vi "CRYStatistics.vi"(0 "Setup in":T1={"No.VI"=0, "Category"="", "StepName"="", "Seq setup flattened"="", "Comment"="", "Steps config."=[], "Jump config"=[], "Start"=0.0, "Increment"=0.0, "Name"="Pa", "Unit"="Pa", "Y data"=1, "Y prefix"="", "Y dB ref"=1.0, "Y unit"="", "Repeat State Array"=[]} {"Repeat State Array"."Start" format="%#_5g"; "Y dB ref" format="%.1f"; "Y data" items=["dB", "Lin"]; "Start" format="%#_5g"}, 5 "Data in":T6 {"Z data" items=["dB", "Lin"]; "X data" items=["dB", "Lin"]; "Y data" items=["dB", "Lin"]; "Z dB ref" format="%.1f"; "Z axis" items=["Log", "Lin"]; "X dB ref" format="%.1f"; "X axis" items=["Log", "Lin"]; "Y axis" items=["Log", "Lin"]; "Y dB ref" format="%.1f"; "Curve"."z" format="%.2f"; "Curve"."y" format="%.2f"; "Curve"."x" format="%.2f"}, 7 "Results in":T2 {"Margin" format="%.2f"}, 9 "Seq Setup in":string, 11 "Step name":string, 12 "Hardware in":string, 13 "Calibration in":string) -> (3 "Types Out":string[](array[string]), 4 "Inserted Names Out":string[](array[string]), 6 "Data out":T6 {"Z data" items=["dB", "Lin"]; "X data" items=["dB", "Lin"]; "Y data" items=["dB", "Lin"]; "Z dB ref" format="%.1f"; "Z axis" items=["Log", "Lin"]; "X dB ref" format="%.1f"; "X axis" items=["Log", "Lin"]; "Y axis" items=["Log", "Lin"]; "Y dB ref" format="%.1f"; "Curve"."z" format="%.2f"; "Curve"."y" format="%.2f"; "Curve"."x" format="%.2f"}, 8 "Results out":T2 {"Margin" format="%.2f"}, 10 "Wave out":T4 {"Y dB ref" format="%.1f"; "Y axis" items=["Log", "Lin"]; "Y data" items=["dB", "Lin"]; "X data" items=["dB", "Lin"]})   [LabVIEW 2013]
uses:
  Typedef Control/CRYData Cluster Array.ctl
  Typedef Control/CRYData Cluster.ctl
  Typedef Control/CRYResult Cluster Array.ctl
  Typedef Control/CRYResult Cluster.ctl
  Typedef Control/CRYWaveform Cluster Array.ctl
  Typedef Control/CRYWaveform Cluster.ctl
  Typedef Control/CRYStep.ctl
  Task Sequence/CRYProject Run Control Global.vi
panel:
  in  "Display Step":bool=TRUE
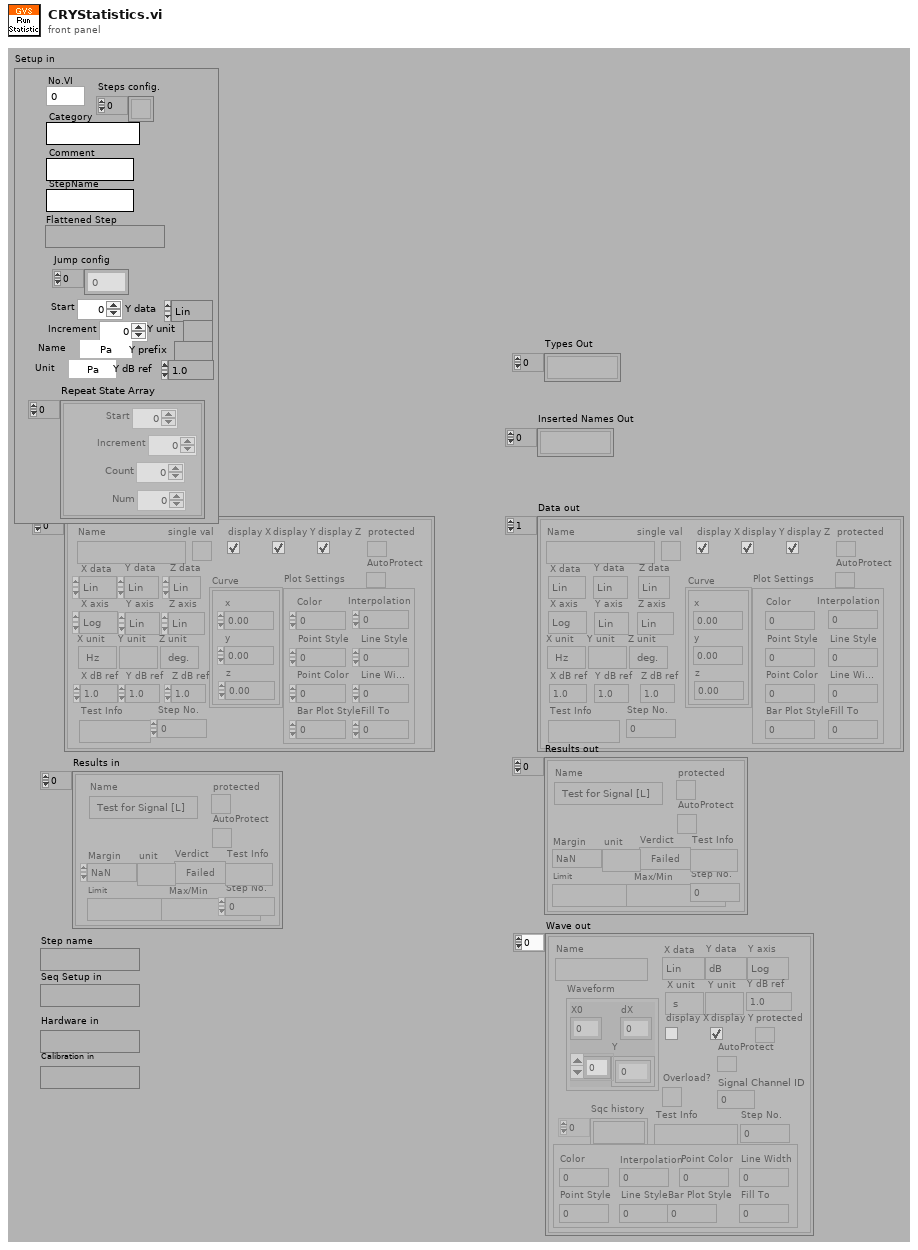
[diagram p1: front panel]
types:
  T1 = typedef "CRYStep.ctl" = cluster{"No.VI":i32, "Category":string, "StepName":string, "Seq setup flattened":string, "Comment":string, "Steps config.":bool[], "Jump config":i32[], "Start":dbl, "Increment":dbl, "Name":string, "Unit":string, "Y data":u16, "Y prefix":string, "Y dB ref":dbl, "Y unit":string, "Repeat State Array":cluster{"Start":dbl, "Increment":dbl, "Count":i32, "Num":i32}[]}
  T2 = typedef "CRYResult Cluster Array.ctl" = T3[]
  T3 = typedef "CRYResult Cluster.ctl" = cluster{"Name":string, "Margin":dbl, "unit":string, "Verdict":bool, "Limit":string, "Max/Min":string, "protected":bool, "Step No.":i32, "Test Info":string, "AutoProtect":bool}
  T4 = typedef "CRYWaveform Cluster Array.ctl" = T5[]
  T5 = typedef "CRYWaveform Cluster.ctl" = cluster{"Waveform":cluster{"X0":dbl, "dX":dbl, "Y":sgl[]}, "X data":u16, "Y data":u16, "Y axis":u16, "X unit":string, "Y unit":string, "Y dB ref":dbl, "display Y":bool, "display X":bool, "Overload?":bool, "Test Info":string, "Step No.":i32, "Name":string, "protected":bool, "Sqc history":string[], "Signal Channel ID":i32, "Plot Settings":cluster{"Color":u32, "Interpolation":u8, "Point Style":u8, "Line Style":u8, "Point Color":u32, "Line Width":u8, "Bar Plot Style":u8, "Fill To":i16}, "AutoProtect":bool}
  T6 = typedef "CRYData Cluster Array.ctl" = T7[]
  T7 = typedef "CRYData Cluster.ctl" = cluster{"Name":string, "Curve":cluster{"x":dbl, "y":dbl, "z":dbl}[], "X data":u16, "Y data":u16, "Z data":u16, "X axis":u16, "Y axis":u16, "Z axis":u16, "X unit":string, "Y unit":string, "Z unit":string, "X dB ref":dbl, "Y dB ref":dbl, "Z dB ref":dbl, "single val":bool, "protected":bool, "display X":bool, "display Y":bool, "display Z":bool, "Test Info":string, "Step No.":i32, "Plot Settings":cluster{"Color":u32, "Interpolation":u8, "Point Style":u8, "Line Style":u8, "Point Color":u32, "Line Width":u8, "Bar Plot Style":u8, "Fill To":i16}, "AutoProtect":bool}
  T8 = cluster{"Start":dbl, "Increment":dbl, "Count":i32, "Num":i32}[]
  T9 = typedef "CRYStatistic cluster.ctl" = cluster{"Mode":u16, "No.Ranked(BF)":i32, "No.Ranked(WF)":i32, "Absolute Margin Standard Deviation":bool, "+/- sigma Res":i32, "Margin Standard Deviation":bool, "Margin Mean":bool, "Overall Yield":bool, "Individual Limits Yield":bool, "LSL Unit":string, "USL Unit\n":string, "LSL":dbl, "USL":dbl, "Worst Fit to Average":bool, "Best Fit to Average":bool, "Ppk":bool, "Pp":bool, "Absolute Standard Deviation":bool, "+/- sigma Dat":i32, "Standard Deviation ":bool, "Mean":bool, "Min ":bool, "Max ":bool, "No.of Curves Selected":i32, "Curves":string[], " Results":string[], "Name":string, "Help":string, "Tab Value":enum32{"Setting", "Help"}, "Work in":u16, "Mode xyz":u16}
  T10 = cluster{"Max ":bool, "Min ":bool, "Mean":bool, "Absolute Standard Deviation":bool, "Standard Deviation ":bool, "Pp":bool, "Ppk":bool, "Best Fit to Average":bool, "Worst Fit to Average":bool}
  T11 = cluster{"Individual Limits Yield":bool, "Overall Yield":bool, "Margin Mean":bool, "Absolute Margin Standard Deviation":bool, "Margin Standard Deviation":bool}
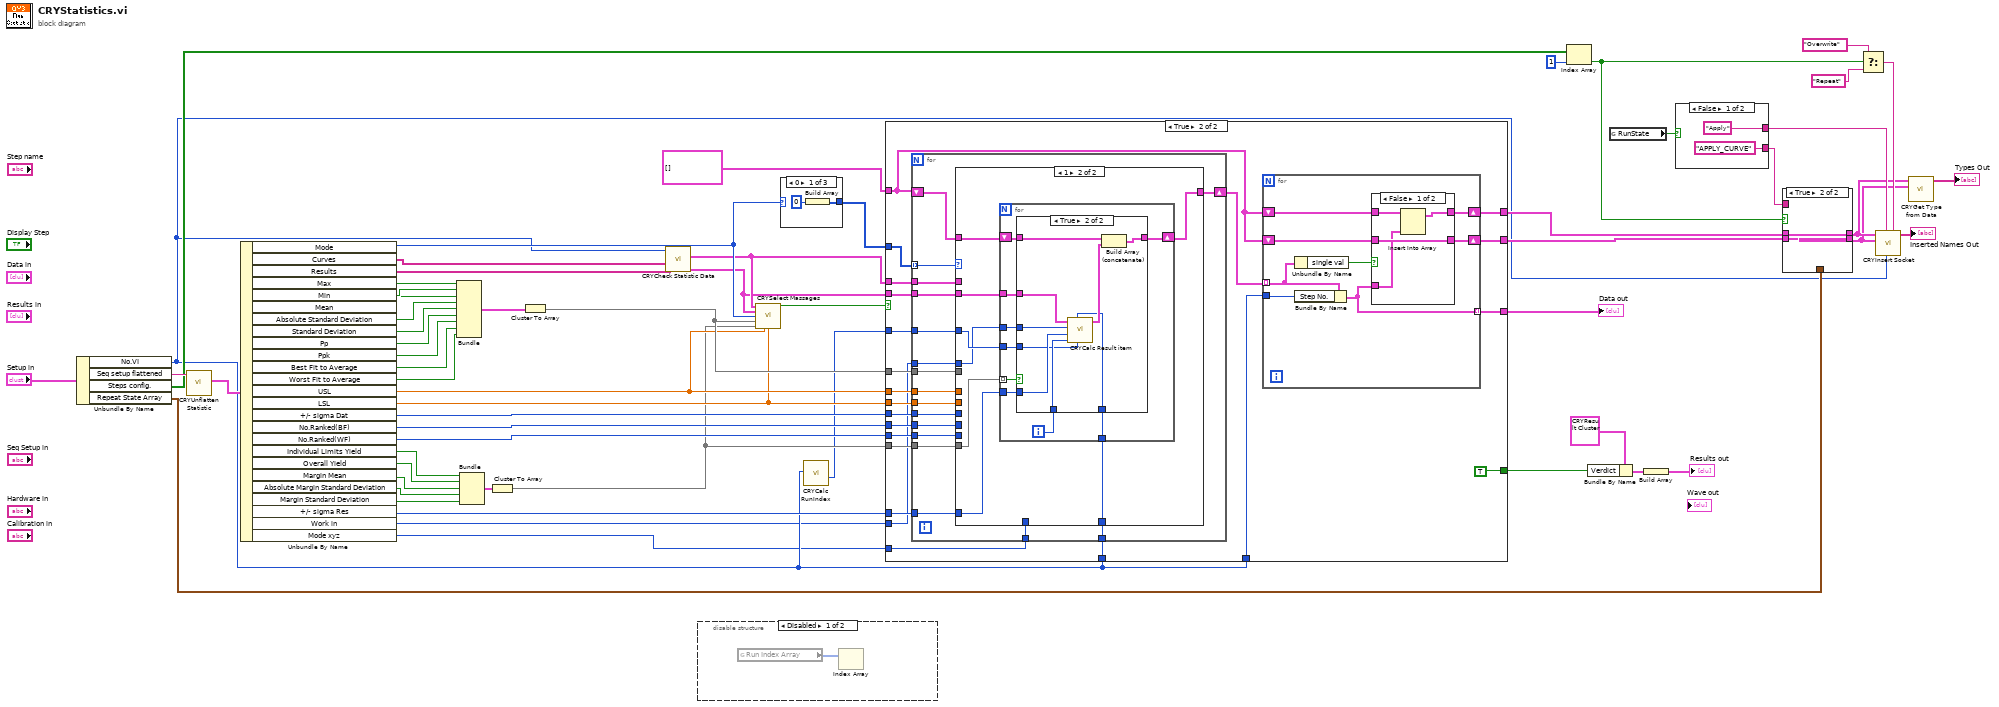
[diagram p0: block diagram]
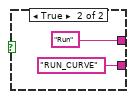
[diagram p3: hidden frame]
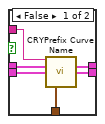
[diagram p4: hidden frame]
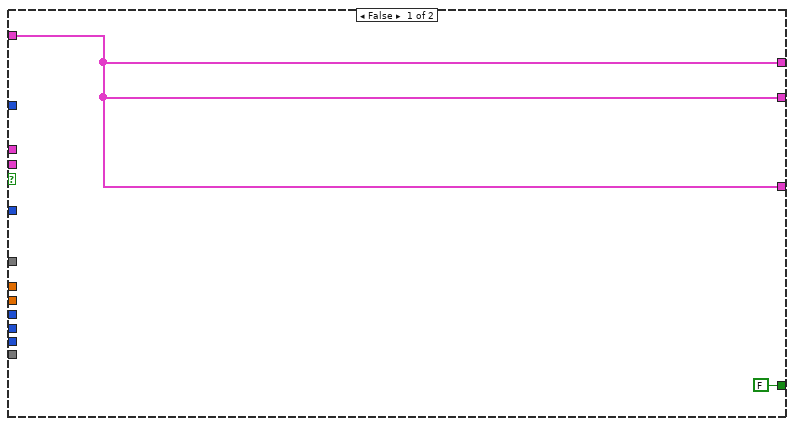
[diagram p5: hidden frame]
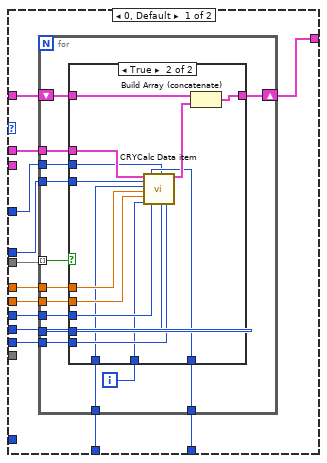
[diagram p6: hidden frame]
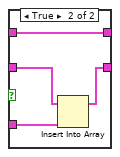
[diagram p9: hidden frame]
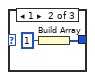
[diagram p10: hidden frame]
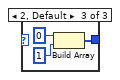
[diagram p11: hidden frame]
diagram:
  n1 = Unbundle By Name("Setup in") -> ("No.VI"=w3:i32, "Seq setup flattened"=w27:string, "Steps config."=w22:bool[], "Repeat State Array"=w17:T8)
  n2 = call "CRYUnflatten Statistic.vi"("Flatten Statistics"=w27) -> ("Statistics"=w29:T9)  [unwired: 10 out]
  n3 = Unbundle By Name(w29) -> ("Mode"=w52:u16, "Curves"=w7:string[], "Results"=w6:string[], "Max"=w44:bool, "Min"=w43:bool, "Mean"=w42:bool, "Absolute Standard Deviation"=w41:bool, "Standard Deviation"=w40:bool, "Pp"=w39:bool, "Ppk"=w38:bool, "Best Fit to Average"=w37:bool, "Worst Fit to Average"=w36:bool, "USL"=w55:dbl, "LSL"=w54:dbl, "+/- sigma Dat"=w60:i32, "No.Ranked(BF)"=w59:i32, "No.Ranked(WF)"=w58:i32, "Individual Limits Yield"=w34:bool, "Overall Yield"=w33:bool, "Margin Mean"=w32:bool, "Absolute Margin Standard Deviation"=w31:bool, "Margin Standard Deviation"=w30:bool, "+/- sigma Res"=w57:i32, "Work in"=w2:u16, "Mode xyz"=w1:u16)
  n4 = Bundle("Max"=w44, "Min"=w43, "Mean"=w42, "Absolute Standard Deviation"=w41, "Standard Deviation"=w40, "Pp"=w39, "Ppk"=w38, "Best Fit to Average"=w37, "Worst Fit to Average"=w36) -> (w45:T10)  [unwired: 1 out]
  n5 = Bundle("Individual Limits Yield"=w34, "Overall Yield"=w33, "Margin Mean"=w32, "Absolute Margin Standard Deviation"=w31, "Margin Standard Deviation"=w30) -> (w35:T11)  [unwired: 1 out]
  n6 = Cluster To Array(cluster=w35) -> (array=w53:bool[])
  n7 = Cluster To Array(cluster=w45) -> (array=w56:bool[])
  n8 = call "CRYCheck Statistic Data.vi"("Results"=w6, "Curves"=w7, "No.VI"=w3) -> ("Result Out"=w4:T3[], "Data Out"=w5:T6)  [unwired: 7 in]
  n9 = disable-structure shown="Disabled" {
    frame Disabled {
      n10 = global read "CRYProject Run Control Global.vi" "Run Index Array"() -> (w61:u32[])
      n11 = Index Array(array=w61) -> ()  [unwired: 1 in, 1 out]
    }
    frame Enabled {
    }
  }
  n12 = call "CRYSelect Massages.vi"("Data in"=w5, "Results in"=w4, "Mode"=w52, "Dat_State"=w56, "Res_state"=w53, "USL"=w55, "LSL"=w54) -> ("Run flag"=w46:bool)  [unwired: 3 in, 5 out]
  n13 = case shown="0" w52 {
    tunnel: [w62 w64 w66] -> w51
    frame 0 {
      n14 = Build Array(0 ("No.Ranked(WF)")) -> (w62:i32[])
    }
    frame 1 {
      n15 = Build Array(1 ("No.Ranked(WF)")) -> (w64:i32[])
    }
    frame 2, Default {
      n16 = Build Array(0 ("No.Ranked(WF)"), 1 ("No.Ranked(WF)")) -> (w66:i32[])
    }
  }
  n17 = call "CRYCalc RunIndex.vi"("No.VI"=w3) -> ("Out Index"=w9:i16)  [unwired: 9 in]
  n18 = case shown="True" w46 {
    tunnel: w60 -> [_ w92]
    tunnel: w59 -> [_ w91]
    tunnel: w58 -> [_ w90]
    tunnel: w57 -> [_ w89]
    tunnel: w56 -> [_ w88]
    tunnel: w55 -> [_ w87]
    tunnel: w54 -> [_ w86]
    tunnel: w53 -> [_ w85]
    tunnel: T6 [] ("Data in") -> [w70 w84]
    tunnel: w5 -> [_ w83]
    tunnel: w4 -> [_ w82]
    tunnel: w3 -> [_ w81]
    tunnel: w51 -> [_ w80]
    tunnel: [w70 w79] -> w47
    tunnel: [w70 w78] -> w20
    tunnel: [w70 w77] -> w19
    tunnel: w3 -> [_ w75]
    tunnel: [FALSE ("Verdict") TRUE ("Verdict")] -> w21
    tunnel: w9 -> [_ w73]
    tunnel: w2 -> [_ w72]
    tunnel: w1 -> [_ w71]
    frame False {
    }
    frame True {
      n19 = for {
        tunnel: w80 -> [w109] mode=indexing
        tunnel: w88 -> [w108]
        tunnel: w85 -> [w107]
        tunnel: w92 -> [w106]
        tunnel: w91 -> [w105]
        tunnel: w90 -> [w104]
        tunnel: w89 -> [w103]
        tunnel: w87 -> [w102]
        tunnel: w86 -> [w101]
        tunnel: w83 -> [w100]
        tunnel: w82 -> [w99]
        shift-right: [w97] -> w76
        shift-left: w84 -> [w98]
        tunnel: w75 -> [w96]
        tunnel: w73 -> [w95]
        tunnel: w72 -> [w94]
        tunnel: w71 -> [w93]
        n20 = case shown="1" w109 {
          tunnel: w108 -> [w122 _]
          tunnel: w107 -> [_ w158]
          tunnel: w106 -> [w121 _]
          tunnel: w105 -> [w118 _]
          tunnel: w104 -> [w117 _]
          tunnel: w103 -> [_ w159]
          tunnel: w102 -> [w120 _]
          tunnel: w101 -> [w119 _]
          tunnel: w100 -> [w116 _]
          tunnel: w99 -> [_ w157]
          tunnel: w98 -> [w115 w156]
          tunnel: [w114 w155] -> w97
          tunnel: w96 -> [w113 w154]
          tunnel: w95 -> [w112 w153]
          tunnel: w94 -> [w111 w152]
          tunnel: w93 -> [w110 _]
          frame 0, Default {
            n21 = for {
              tunnel: w122 -> [w132] mode=indexing
              tunnel: w121 -> [w136]
              tunnel: w120 -> [w135]
              tunnel: w119 -> [w134]
              tunnel: w118 -> [w131]
              tunnel: w117 -> [w133]
              tunnel: w116 -> [w129]
              shift-right: [w127] -> w114
              shift-left: w115 -> [w128]
              tunnel: w113 -> [w126]
              tunnel: w112 -> [w125]
              tunnel: w111 -> [w124]
              tunnel: w110 -> [w123]
              i -> [w130]
              n22 = case shown="True" w132 {
                tunnel: w130 -> [_ w148]
                tunnel: w136 -> [_ w151]
                tunnel: w135 -> [_ w147]
                tunnel: w134 -> [_ w146]
                tunnel: w131 -> [_ w150]
                tunnel: w133 -> [_ w149]
                tunnel: w129 -> [_ w142]
                tunnel: [w137 w143] -> w127
                tunnel: w128 -> [w137 w145]
                tunnel: w126 -> [_ w141]
                tunnel: w125 -> [_ w140]
                tunnel: w124 -> [_ w139]
                tunnel: w123 -> [_ w138]
                frame False {
                }
                frame True {
                  n23 = call "CRYCalc Data item.vi"("Data in"=w142, "Work in"=w139, "Mode xyz"=w138, "USL"=w147, "LSL"=w146, "Statistic Item"=w148, "Step Setup VI No"=w141, "+/-Adjust(Deviation)"=w151, "Statistic Run Number"=w140, "rank number(best curve)"=w150, "rank number(worst curve)"=w149) -> ("Data out"=w144:T6)  [unwired: 8 in]
                  n24 = Build Array (concatenate)(w145, w144) -> (w143:T6)
                }
              }
            }
          }
          frame 1 {
            n25 = for {
              tunnel: w158 -> [w168] mode=indexing
              tunnel: w159 -> [w167]
              tunnel: w157 -> [w165]
              shift-right: [w163] -> w155
              shift-left: w156 -> [w164]
              tunnel: w154 -> [w162]
              tunnel: w153 -> [w161]
              tunnel: w152 -> [w160]
              i -> [w166]
              n26 = case shown="True" w168 {
                tunnel: w166 -> [_ w176]
                tunnel: w167 -> [_ w177]
                tunnel: w165 -> [_ w178]
                tunnel: w164 -> [w169 w175]
                tunnel: [w169 w173] -> w163
                tunnel: w162 -> [_ w172]
                tunnel: w161 -> [_ w171]
                tunnel: w160 -> [_ w170]
                frame False {
                }
                frame True {
                  n27 = call "CRYCalc Result item.vi"("Statistic Run Number"=w171, "Step Setup VI No"=w172, "Statistic Item"=w176, "+/-Adjust(Deviation)"=w177, "Work in"=w170, "Results in"=w178) -> ("Result  run Out"=w174:T7[])  [unwired: 4 out]
                  n28 = Build Array (concatenate)(w175, w174) -> (w173:T6)
                }
              }
            }
          }
        }
      }
      n29 = for {
        tunnel: w76 -> [w186] mode=indexing
        tunnel: w81 -> [w185]
        tunnel: [w183] -> w79 mode=indexing
        shift-right: [w181] -> w77
        shift-left: w84 -> [w182]
        shift-right: [w179] -> w78
        shift-left: w84 -> [w180]
        n30 = Unbundle By Name(w186) -> ("single val"=w184:bool)
        n31 = Bundle By Name(cluster=w186, "Step No."=w185) -> (w183:T7)
        n32 = case shown="False" w184 {
          tunnel: w183 -> [w187 w191]
          tunnel: w182 -> [w188 w194]
          tunnel: [w188 w193] -> w181
          tunnel: w180 -> [w190 w192]
          tunnel: [w189 w192] -> w179
          frame False {
            n33 = Insert Into Array(array=w190, new element=w187) -> (w189:T6)  [unwired: 1 in]
          }
          frame True {
            n34 = Insert Into Array(array=w194, new element=w191) -> (w193:T6)  [unwired: 1 in]
          }
        }
      }
    }
  }
  "Data out" <- w47
  n35 = Index Array(array=w22, index=1) -> (element=w18:bool)
  n36 = Bundle By Name(cluster=T3 {"Name"="Test for Signal [L]", "Margin"=nan, "unit"="", "Verdict"=FALSE, "Limit"="", "Max/Min"="", "protected"=FALSE, "Step No."=0, "Test Info"="", "AutoProtect"=FALSE} ("Result"), "Verdict"=w21) -> (w49:T3)
  n37 = global read "CRYProject Run Control Global.vi" "RunState"() -> (w16:bool)
  n38 = Build Array(w49) -> (→"Results out":T3[])
  n39 = case shown="False" w16 {
    tunnel: ["Apply" ("sOption1") "Run" ("Type In")] -> w15
    tunnel: ["APPLY_CURVE" ("Type In") "RUN_CURVE" ("Type In")] -> w14
    frame False {
    }
    frame True {
    }
  }
  n40 = case shown="True" w18 {
    tunnel: w20 -> [w204 w206]
    tunnel: w19 -> [w203 w205]
    tunnel: [w202 w206] -> w11
    tunnel: [w201 w205] -> w10
    tunnel: w17 -> [w200 _]
    tunnel: w14 -> [w199 _]
    frame False {
      n41 = call "CRYPrefix Curve Name.vi"("Type In"=w199, "Curves In"=w204, "Values In"=w203, "Repeat State Array In"=w200) -> ("Curves Out"=w202:T6, "Values Out"=w201:T6)  [unwired: 8 in, 2 out]
    }
    frame True {
    }
  }
  n42 = Select(t="Overwrite" ("Y unit"), s=w18, f="Repeat") -> (s? t:f=w23:string)
  n43 = call "CRYInsert Socket.vi"("sOption2"=w23, "Step No."=w3, "sOption1"=w15, "Values"=w10, "Curves"=w11) -> ("Inserted Names Out"=→"Inserted Names Out":string[])  [unwired: 6 in]
  n44 = call "CRYGet Type from Data.vi"("Values"=w10, "Curves"=w11) -> ("Type"=→"Types Out":string[])  [unwired: 9 in]
